vi "time_get_unix.vi"() -> (0 "unix_timestamp":dbl format="%.6f")   [LabVIEW 2018]
panel:
  # "Returns UNIX time in seconds"
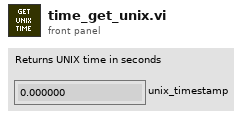
[diagram p1: front panel]
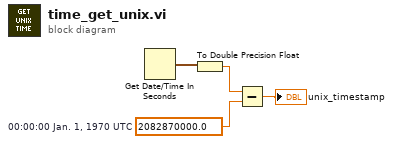
[diagram p0: block diagram]
diagram:
  w1 = 2082870000.0  # 00:00:00 Jan. 1, 1970 UTC
  n1 = Get Date/Time In Seconds() -> (seconds since 1Jan1904=w2:timestamp)
  n2 = To Double Precision Float(number=w2) -> (double precision float=w3:dbl)
  n3 = Subtract(x=w3, y=w1) -> (x-y=→"unix_timestamp":dbl)
